vi "Q14070-B020调整螺塞压装防尘封.vi"() -> ()   [LabVIEW 2013]
uses:
  PCI8622_32.dll
panel:
  out "涂脂工步号":dbl
  out "涂脂报警提示":string
  out "换向力":dbl=2000.0 format="%#_13g"
  out "数值":i32
  out "员工ID":string
  out "型号数量":i32=10
  out "error out 4":errorcluster
  out "B020状态正常":bool
  out "B020有不合格项":bool
  out "报警提示":string
  in  "员工权限":bool=TRUE
  out "点胶工步号":dbl
  out "点胶操作状态":string
  out "涂脂操作状态":string
  out "涂脂工步号":dbl
  out "压装操作状态":string
  in  "联线按钮":bool
  out "电动缸位置(mm)":dbl format="%#_3f"
  in  "压装工步号":dbl
  out "调整螺塞压头压力(N)":dbl format="%#.1f"
  out "调整螺塞压头位移(mm)":dbl format="%#.3f"
  out "通讯状态":bool
  in  "停止":bool
  in  "选项卡控件 2":enum32{"自动", "手动", "传感器校验", "参数查询"}(tab)
  out "防尘封压装最大力(N)":dbl
  out "区域压力最大值(N)":dbl format="%#_4g"
  out "区域压力最小值(N)":dbl format="%#_4g"
  in  "压装不合格提示按钮":bool
  out "调整螺塞压防尘封":cluster{dbl[], dbl[]}[](graph)
  out "压装合格":bool
  out "压装不合格":bool
  out "压装位移(mm)":dbl format="%#_4g"
  out "监控点压力(N)":dbl format="%#_4g"
  in  "电动缸速度(s/mm)":dbl
  out "当前位置":dbl
  in  "电动缸手动位置(mm)":dbl
  in  "?":bool
  in  "防尘封涂脂":bool
  in  "手动点胶关":bool
  out "防尘封在位检测":bool
  out "涂脂在位":bool
  out "点胶在位":bool
  out "光幕":bool
  out "电动缸报警":bool
  out "电动缸原点检测":bool
  out "电动缸正极限":bool
  out "电动缸负极限":bool
  in  "M光幕无效按钮":bool
  in  "电机停止":bool
  in  "电机下降":bool
  in  "电机上升":bool
  in  "电机复位":bool
  in  "电机回原点":bool
  in  "电机使能开":bool
  in  "手动点胶开":bool
  in  "调整螺塞涂脂":bool
  in  "涂脂单循环":bool
  in  "压装单循环":bool
  in  "点胶单循环":bool
  in  "位移传感器零点偏移":dbl format="%#.2f"
  in  "位移传感器比例偏移":dbl format="%#.2f"
  in  "压力传感器零点偏移":dbl format="%#.2f"
  in  "压力传感器比例偏移":dbl format="%#.2f"
  in  "传感器参数查询":bool
  in  "传感器参数保存":bool
  in  "参数查询":bool
  in  "参数列表":string[][](table)
  in  "参数修改":bool
  out "员工姓名":string
  in  "型号选择":u16(ring) items=["J709", "J728", "J706"]
  in  "参数加载":bool
  out "报警工步号":dbl
  out "error out":errorcluster
  out "error out 2":errorcluster
  out "区域最大位移1(mm)":dbl format="%#.1f"
  out "区域最小位移1(mm)":dbl format="%#.1f"
  out "区域最大压力1(KN)":dbl format="%#.3f"
  out "位移监控点1(mm)":dbl format="%#.1f"
  out "监控点最小压力1(KN)":dbl format="%#.3f"
  out "监控点最大压力1(KN)":dbl format="%#.3f"
  out "最小压入位移1(mm)":dbl format="%#.1f"
  out "最大压入位移1(mm)":dbl format="%#.1f"
  out "区域最小压力1(KN)":dbl format="%#.3f"
  out "区域最小压力2(KN)":dbl format="%#.3f"
  out "最小压入位移2(mm)":dbl format="%#.1f"
  out "最大压入位移2(mm)":dbl format="%#.1f"
  out "区域最大压力2(KN)":dbl format="%#.3f"
  out "位移监控点2(mm)":dbl format="%#.1f"
  out "监控点最大压力2(KN)":dbl format="%#.3f"
  out "监控点最小压力2(KN)":dbl format="%#.3f"
  out "区域最小位移2(mm)":dbl format="%#.1f"
  out "区域最大位移2(mm)":dbl format="%#.1f"
  out "伺服1快进位置设置":dbl format="%#.1f"
  out "伺服1慢进位置设置":dbl format="%#.1f"
  out "压装涂脂设定次数":dbl
  out "涂脂1设定次数":dbl
  out "伺服1快进速度设置":dbl format="%#.1f"
  out "ADODB._Connection Out":refnum<k7>
  out "error out 3":errorcluster
  # "芜湖机械转向器装配线"
  # "调整螺塞压装防尘封"
  # "湖北唯思凌科装备制造有限公司 设计开发 (C)2015"
  # "Q14070机械转向器装配线"
  # "传感器校验区"
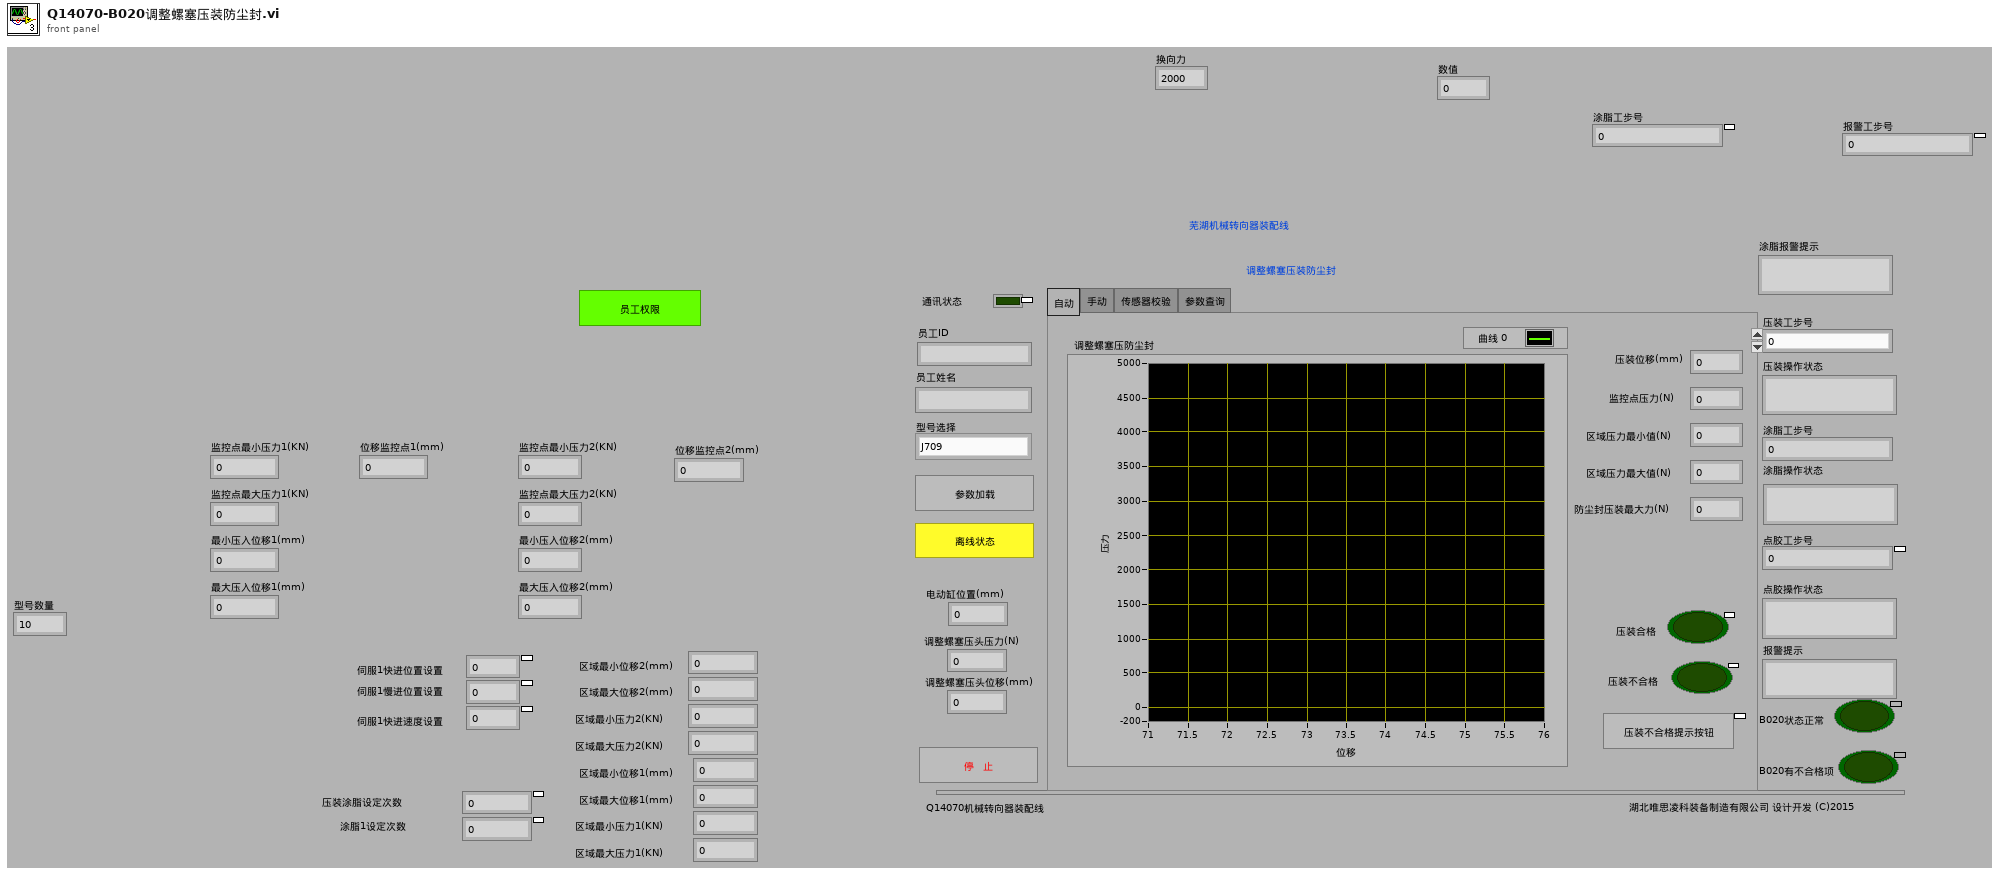
[diagram p1: front panel]
types:
  T1 = typedef "imagedata.ctl" = cluster{"image type":i32, "image depth":i32, "image":u8[], "mask":u8[], "colors":u32[], "Rectangle":cluster{"left":i16, "top":i16, "right":i16, "bottom":i16}}
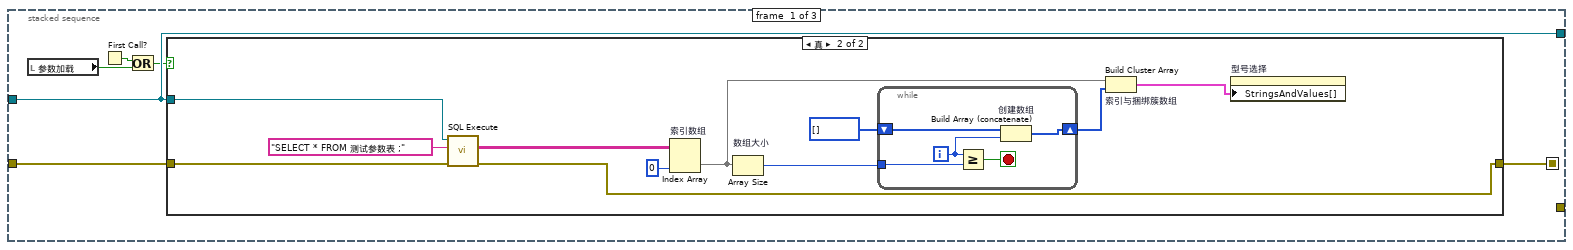
[diagram p3: hidden frame]
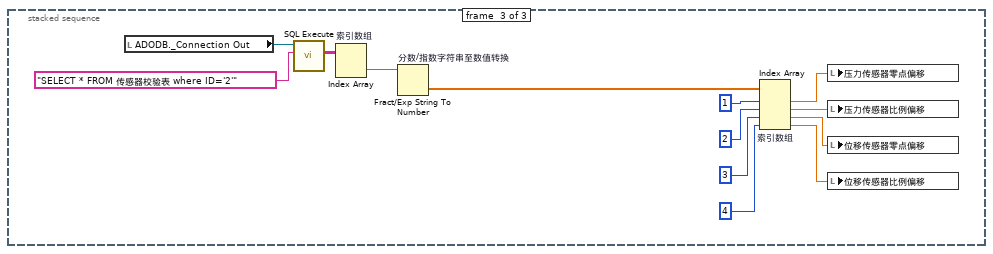
[diagram p5: hidden frame]
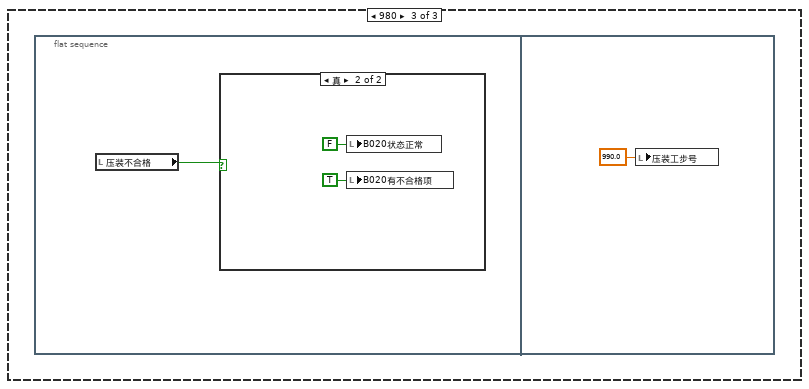
[diagram p8: hidden frame]
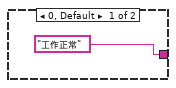
[diagram p10: hidden frame]
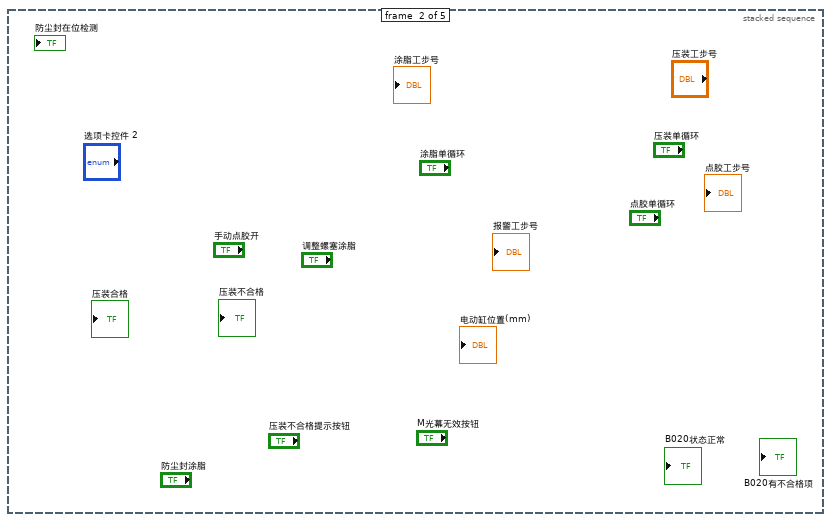
[diagram p11: hidden frame]
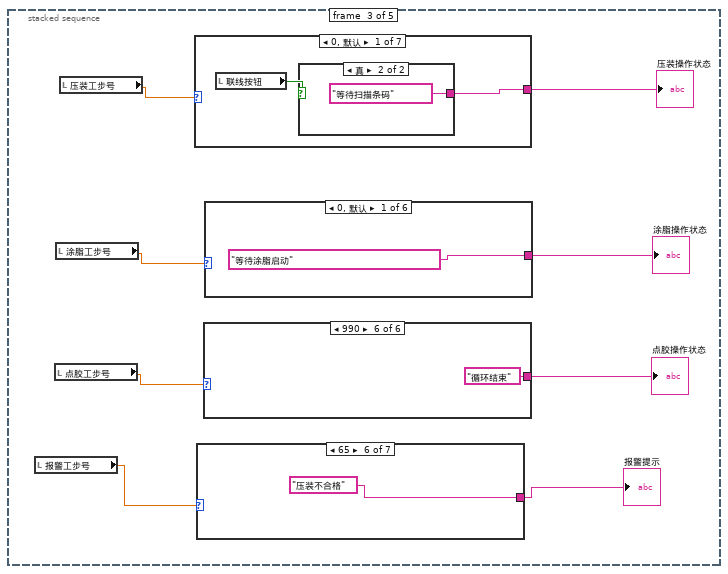
[diagram p12: hidden frame]
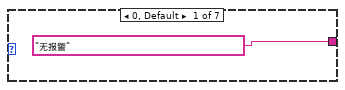
[diagram p13: hidden frame]
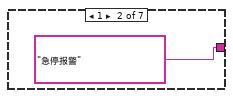
[diagram p14: hidden frame]
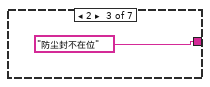
[diagram p15: hidden frame]
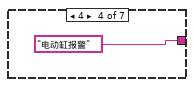
[diagram p16: hidden frame]
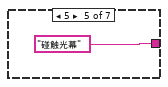
[diagram p17: hidden frame]
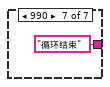
[diagram p18: hidden frame]
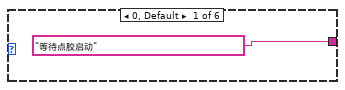
[diagram p19: hidden frame]
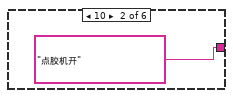
[diagram p20: hidden frame]
diagram:
  n1 = while {
    stop <- w8 stop-if-true
    n2 = event shown="[1] \"参数查询\": 值改变" {
      selector: _ -> [_ _ _ _ _]
      dyn-events: _ -> [_ _ _ _ _]
      timeout: 500 -> [_ _ _ _ _]
      event Timeout {
        n3 = event-data() -> ()  [unwired: 3 out]
      }
      event "参数查询": Value Change {
        n4 = event-data() -> ()  [unwired: 7 out]
        n5 = flat-sequence {
          tunnel: [w19] -> w16
          tunnel: [w29] -> w15
          tunnel: [w25] -> w13
          tunnel: [w22] -> w11
          tunnel: w16 -> [w34]
          tunnel: w15 -> [w32]
          tunnel: [w33] -> w14
          tunnel: w13 -> [w33]
          tunnel: [w32] -> w12
          tunnel: w11 -> [w31]
          tunnel: w14 -> [w37]
          tunnel: w12 -> [w36]
          frame #0 {
            n6 = call "字符串转换为数组.vi"("查询内容"=",产品型号,区域最小位移1,区域最大位移1,区域最小压力1,区域最大压力1,最小压入位移1,最大压入位移1,监控点最小压力1,监控点最大压力1,位移监控点1,区域最小位移2,区域最大位移2,区域最小压力2,区域最大压力2,最小压入位移2,最大压入位移2,监控点最小压力2,监控点最大压力2,位移监控点2,伺服1快进位置设置,伺服1快进速度设置,伺服1慢进位置设置,涂脂1设定次数,压装涂脂设定次数,换向压力") -> ("列首"=w17:string[])  [unwired: 10 in]
            n7 = property on="参数列表" class="Tbl (严格)"("Row Headers[]"=w17) -> ()  [unwired: 2 in, 2 out]
          }
          frame #1 {
            n8 = call "创建文本"() -> ("Result"=w30:string)  [unwired: 14 in, 1 out]
            n9 = call "ADO Connection Create.vi"() -> ("error out"=w24:errorcluster, "ADODB._Connection Out"=w28:refnum<k7>)  [unwired: 10 in]
            n10 = call "ADO Connection Open.vi"("error in (no error)"=w24, "ConnectionString"="DSN=参数B020;", "ADODB._Connection In"=w28) -> ("error out"=w23:errorcluster, "ADODB._Connection Out"=w26:refnum<k7>)  [unwired: 7 in]
            n11 = call "SQL Execute.vi"("error in (no error)"=w23, "Command Text"=w30, "ADODB._Connection In"=w26) -> ("error out"=w29:errorcluster, "Data"=w21:string[][], "ADODB._Connection Out"=w25:refnum<k7>)  [unwired: 5 in, 1 out]
            n12 = Transpose 2D Array "二维数组转置"(2D array=w21) -> (transposed array=w19:string[][])
            n13 = Index Array(array=w19, index (row)=0 ("索引 (行)")) -> (element=w22:string[])  [unwired: 1 in]
          }
          frame #2 {
            n14 = local write "参数列表"(w34) -> ()
            n15 = property on="参数列表" class="Tbl (严格)"("Column Headers[]"=w31) -> ()  [unwired: 2 in, 2 out]
          }
          frame #3 {
            n16 = call "ADO Connection Close.vi"("error in (no error)"=w36, "ADODB._Connection In"=w37) -> ("error out"=→"error out":errorcluster)  [unwired: 8 in, 1 out]
          }
        }
      }
      event "传感器参数保存": Value Change {
        n17 = event-data() -> ()  [unwired: 7 out]
        n18 = local read "压力传感器零点偏移"() -> (w41:dbl)
        n19 = local read "压力传感器比例偏移"() -> (w40:dbl)
        n20 = local read "位移传感器零点偏移"() -> (w39:dbl)
        n21 = local read "位移传感器比例偏移"() -> (w38:dbl)
        n22 = call "ADO Connection Create.vi"() -> ("error out"=w54:errorcluster, "ADODB._Connection Out"=w56:refnum<k7>)  [unwired: 10 in]
        n23 = Number To Fractional String(number=w41, precision (6)=i16 3 ("精度(6)")) -> (F-format string=w47:string)  [unwired: 2 in]
        n24 = Number To Fractional String(number=w40, precision (6)=i16 2 ("精度(6)")) -> (F-format string=w46:string)  [unwired: 2 in]
        n25 = Number To Fractional String(number=w39, precision (6)=i16 1 ("精度(6)")) -> (F-format string=w45:string)  [unwired: 2 in]
        n26 = Number To Fractional String(number=w38, precision (6)=i16 2 ("精度(6)")) -> (F-format string=w44:string)  [unwired: 2 in]
        n27 = call "创建文本2"("位移1比例偏移值"=w44, "压力1零点偏移值"=w47, "压力1比例偏移值"=w46, "位移1零点偏移值"=w45) -> ("Result"=w43:string)  [unwired: 10 in, 1 out]
        n28 = call "ADO Connection Open.vi"("error in (no error)"=w54, "ConnectionString"="DSN=参数B020;", "ADODB._Connection In"=w56) -> ("error out"=w53:errorcluster, "ADODB._Connection Out"=w55:refnum<k7>)  [unwired: 7 in]
        n29 = call "SQL Execute.vi"("error in (no error)"=w53, "Command Text"=w43, "ADODB._Connection In"=w55) -> ("error out"=w57:errorcluster, "ADODB._Connection Out"=w58:refnum<k7>)  [unwired: 5 in, 2 out]
        n30 = call "ADO Connection Close.vi"("error in (no error)"=w57, "ADODB._Connection In"=w58) -> ("error out"=→"error out 3":errorcluster)  [unwired: 8 in, 1 out]
      }
      event "停止": Value Change {
        n31 = event-data() -> ()  [unwired: 7 out]
        n32 = flat-sequence {
          frame #0 {
            n33 = local write "涂脂工步号"(0.0 ("工步号")) -> ()
          }
          frame #1 {
            n34 = Wait Until Next ms Multiple(millisecond multiple=u32 1000 ("毫秒倍数")) -> ()  [unwired: 1 out]
          }
          frame #2 {
            n35 = Quit LabVIEW(quit? (T)=TRUE ("停止？(T)")) -> ()
          }
        }
      }
      event "参数修改": Value Change {
        n36 = event-data() -> ()  [unwired: 7 out]
        n37 = while {
          i -> [w70]
          stop <- w69 stop-if-true
          (unwired) "UPDATE 测试参数表 SET 区域最小位移1='%区域最小位移1%',区域最大位移1='%区域最大位移1%',区域最小压力1='%区域最小压力1%',区域最大压力1='%区域最大压力1%', 最小压入位移1='%最小压入位移1%', 最大压入位移1='%最大压入位移1%',监控点最小压力1='%监控点最小压力1%',监控点最大压力1='%监控点最大压力1%',位移监控点1='%位移监控点1%', 区域最小位移2='%区域最小位移2%' ,区域最大位移2='%区域最大位移2%' ,区域最小压力2='%区域最小压力2%',区域最大压力2='%区域最大压力2%' ,最小压入位移2='%最小压入位移2%' ,最大压入位移2='%最大压入位移2%' ,监控点最小压力2='%监控点最小压力2%' ,监控点最大压力2='%监控点最大压力2%' ,位移监控点2='%位移监控点2%' ,伺服1快进位置设置='%伺服1快进位置设置%' ,伺服1快进速度设置='%伺服1快进速度设置%' ,伺服1慢进位置设置='%伺服1慢进位置设置%' ,伺服1慢进速度设置='%伺服1慢进速度设置%', 涂脂1设定次数='%涂脂1设定次数%'WHERE 产品型号 = '%产品型号%';"
          n38 = local read "参数列表"() -> (w72:string[][])
          n39 = local read "型号数量"() -> (w71:i32)
          n40 = Wait Until Next ms Multiple(millisecond multiple=u32 50 ("毫秒倍数")) -> ()  [unwired: 1 out]
          n41 = Greater Or Equal?(x=w70, y=w71) -> (x >= y?=w69:bool)
          n42 = Index Array(array=w72, index (col)=w70) -> (element=w68:string[])  [unwired: 1 in]
          n43 = stacked-sequence {
            seq-local: [w74 _] -> [_ w122]
            tunnel: w68 -> [w110 w129]
            tunnel: [_ w123] -> w62
            frame #0 {
              n44 = Index Array(array=w110, index #1=1 ("索引"), index #2=2 ("索引"), index #3=3 ("索引"), index #4=4 ("索引"), index #5=5 ("索引"), index #6=6 ("索引"), index #7=7 ("索引"), index #8=8 ("索引"), index #9=9 ("索引"), index #10=10 ("索引"), index #11=11 ("索引"), index #12=12 ("索引"), index #13=13 ("索引"), index #14=14 ("索引"), index #15=15 ("索引"), index #16=16 ("索引"), index #17=17 ("索引"), index #18=18 ("索引"), index #19=19 ("索引"), index #20=20 ("索引"), index #21=21 ("索引"), index #22=22 ("索引"), index #23=23 ("索引")) -> (element #1=w97:string, element #2=w96:string, element #3=w95:string, element #4=w94:string, element #5=w93:string, element #6=w92:string, element #7=w91:string, element #8=w90:string, element #9=w89:string, element #10=w88:string, element #11=w87:string, element #12=w86:string, element #13=w85:string, element #14=w84:string, element #15=w83:string, element #16=w82:string, element #17=w81:string, element #18=w80:string, element #19=w79:string, element #20=w78:string, element #21=w77:string, element #22=w76:string, element #23=w75:string)  [unwired: 1 in, 1 out]
              n45 = call "创建文本6"("区域最小位移1"=w97, "区域最大位移1"=w96, "区域最小压力1"=w95, "区域最大压力1"=w94, "最小压入位移1"=w93, "最大压入位移1"=w92, "监控点最小压力1"=w91, "监控点最大压力1"=w90, "位移监控点1"=w89, "区域最小位移2"=w88, "区域最大位移2"=w87, "区域最小压力2"=w86, "区域最大压力2"=w85, "最小压入位移2"=w84, "最大压入位移2"=w83, "监控点最小压力2"=w82, "监控点最大压力2"=w81, "位移监控点2"=w80, "伺服1快进位置设置"=w79, "伺服1快进速度设置"=w78, "伺服1慢进位置设置"=w77, "涂脂1设定次数"=w76, "压装涂脂设定次数"=w75) -> ("Result"=w74:string)  [unwired: 3 in, 1 out]
            }
            frame #1 {
              n46 = Index Array(array=w129, index #1=24, index #2=0) -> (element #1=w126:string, element #2=w125:string)  [unwired: 6 in, 6 out]
              n47 = call "创建文本5"("换向压力"=w126, "产品型号"=w125) -> ("Result"=w124:string)  [unwired: 12 in, 1 out]
              n48 = Concatenate Strings(w122, w124) -> (w123:string)
            }
          }
          n49 = local read "ADODB._Connection Out"() -> (w64:refnum<k7>)
          n50 = call "SQL Execute.vi"("error in (no error)"=errorcluster {"status"=FALSE, "code"=0, "source"=""}, "Command Text"=w62, "ADODB._Connection In"=w64) -> ("error out"=w66:errorcluster, "ADODB._Connection Out"=w67:refnum<k7>)  [unwired: 5 in, 2 out]
          n51 = call "ADO Connection Close.vi"("error in (no error)"=w66, "ADODB._Connection In"=w67) -> ("error out"=→"error out 4":errorcluster)  [unwired: 8 in, 1 out]
        }
      }
    }
    n52 = Wait Until Next ms Multiple(millisecond multiple=u32 50 ("毫秒倍数")) -> ()  [unwired: 1 out]
    n53 = local read "停止"() -> (w8:bool)
  }
  n54 = flat-sequence {
    tunnel: [w131] -> w4
    tunnel: [w130] -> w3
    tunnel: w4 -> [w138]
    tunnel: w3 -> [w137]
    tunnel: [w136] -> w2
    tunnel: [w135] -> w1
    tunnel: w2 -> [w248]
    tunnel: w1 -> [w247]
    frame #0 {
      n55 = call "ADO Connection Create.vi"() -> ("error out"=w133:errorcluster, "ADODB._Connection Out"=w134:refnum<k7>)  [unwired: 10 in]
      n56 = call "ADO Connection Open.vi"("error in (no error)"=w133, "ConnectionString"="DSN=参数B020;", "ADODB._Connection In"=w134) -> ("error out"=w130:errorcluster, "ADODB._Connection Out"=w131:refnum<k7>)  [unwired: 7 in]
      "ADODB._Connection Out" <- w131
    }
    frame #1 {
      n57 = while {
        tunnel: w138 -> [w143]
        tunnel: w137 -> [w142]
        tunnel: [w141] -> w136
        tunnel: [w140] -> w135
        stop <- w146 stop-if-true
        n58 = local read "参数加载"() -> (w139:bool)
        n59 = Wait (ms)(milliseconds to wait=u32 100 ("等待时间（毫秒）")) -> ()  [unwired: 1 out]
        n60 = First Call?() -> (First Call?: T/F=w145:bool)
        n61 = Or(x=w145, y=w139) -> (x .or. y?=w144:bool)
        n62 = case shown="真" w144 {
          tunnel: w143 -> [w149 w153]
          tunnel: w142 -> [w148 w152]
          tunnel: [w149 w151] -> w141
          tunnel: [w148 w150] -> w140
          frame False {
          }
          frame True {
            n63 = stacked-sequence {
              seq-local: [w157 _ _] -> [_ w231 _]
              tunnel: w153 -> [w158 w228 _]
              tunnel: w152 -> [w159 _ _]
              tunnel: [w158 _ _] -> w151
              tunnel: [_ w230 _] -> w150
              frame #0 {
                n64 = local read "参数加载"() -> (w155:bool)
                n65 = First Call?() -> (First Call?: T/F=w156:bool)
                n66 = Or(x=w156, y=w155) -> (x .or. y?=w154:bool)
                n67 = case shown="真" w154 {
                  tunnel: w159 -> [w160 w165]
                  tunnel: w158 -> [_ w163]
                  tunnel: [w160 w162] -> w157
                  frame False {
                  }
                  frame True {
                    n68 = call "SQL Execute.vi"("error in (no error)"=w165, "Command Text"="SELECT * FROM 测试参数表 ;", "ADODB._Connection In"=w163) -> ("error out"=w162:errorcluster, "Data"=w166:string[][])  [unwired: 5 in, 2 out]
                    n69 = Index Array "索引数组"(array=w166, index (col)=0 ("禁用的索引 (列)")) -> (element=w169:string[])  [unwired: 1 in]
                    n70 = Array Size "数组大小"(array=w169) -> (size(s)=w168:i32)
                    n71 = while {
                      shift-right: [w174] -> w167
                      shift-left: i32[] [] -> [w175]
                      tunnel: w168 -> [w172]
                      i -> [w173]
                      stop <- w176 stop-if-true
                      n72 = Greater Or Equal?(x=w173, y=w172) -> (x >= y?=w176:bool)
                      n73 = Build Array (concatenate) "创建数组"(w175, w173) -> (w174:i32[])
                    }
                    n74 = Build Cluster Array "索引与捆绑簇数组"(w169, w167) -> (w161:cluster{"String":string, i32}[])
                    n75 = property on="型号选择" class="Ring (严格)"("StringsAndValues[]"=w161) -> ()  [unwired: 2 in, 2 out]
                  }
                }
              }
              frame #1 {
                n76 = property on="型号选择" class="Ring (严格)"() -> ("RingText.Text"=w227:string)  [unwired: 2 in, 2 out]
                n77 = call "创建文本4"("产品型号"=w227) -> ("Result"=w229:string)  [unwired: 13 in, 1 out]
                n78 = call "SQL Execute.vi"("error in (no error)"=w231, "Command Text"=w229, "ADODB._Connection In"=w228) -> ("error out"=w230:errorcluster, "Data"=w233:string[][])  [unwired: 5 in, 2 out]
                n79 = Index Array "索引数组"(array=w233, index (row)=0 ("索引 (行)")) -> (element=w226:string[])  [unwired: 1 in]
                n80 = Fract/Exp String To Number "分数/指数字符串至数值转换"(string=w226) -> (number=w181:dbl[])  [unwired: 3 in, 1 out]
                n81 = Index Array(array=w181, index #1=1 ("索引"), index #2=2 ("索引"), index #3=3 ("索引"), index #4=4 ("索引"), index #5=5 ("索引"), index #6=6 ("索引"), index #7=7 ("索引"), index #8=8 ("索引"), index #9=9 ("索引"), index #10=10 ("索引"), index #11=11 ("索引"), index #12=12 ("索引"), index #13=13 ("索引"), index #14=14 ("索引"), index #15=15 ("索引"), index #16=16 ("索引"), index #17=17 ("索引"), index #18=18 ("索引"), index #19=19 ("索引"), index #20=20 ("索引"), index #21=21 ("索引"), index #22=22 ("索引"), index #23=23 ("索引"), index #24=24 ("索引")) -> (element #1=→"区域最小位移1(mm)":dbl, element #2=→"区域最大位移1(mm)":dbl, element #3=→"区域最小压力1(KN)":dbl, element #4=→"区域最大压力1(KN)":dbl, element #5=→"最小压入位移1(mm)":dbl, element #6=→"最大压入位移1(mm)":dbl, element #7=→"监控点最小压力1(KN)":dbl, element #8=→"监控点最大压力1(KN)":dbl, element #9=→"位移监控点1(mm)":dbl, element #10=→"区域最小位移2(mm)":dbl, element #11=→"区域最大位移2(mm)":dbl, element #12=→"区域最小压力2(KN)":dbl, element #13=→"区域最大压力2(KN)":dbl, element #14=→"最小压入位移2(mm)":dbl, element #15=→"最大压入位移2(mm)":dbl, element #16=→"监控点最小压力2(KN)":dbl, element #17=→"监控点最大压力2(KN)":dbl, element #18=→"位移监控点2(mm)":dbl, element #19=→"伺服1快进位置设置":dbl, element #20=→"伺服1快进速度设置":dbl, element #21=→"伺服1慢进位置设置":dbl, element #22=→"涂脂1设定次数":dbl, element #23=→"压装涂脂设定次数":dbl, element #24=→"换向力":dbl)
              }
              frame #2 {
                n82 = local read "ADODB._Connection Out"() -> (w241:refnum<k7>)
                n83 = call "SQL Execute.vi"("Command Text"="SELECT * FROM 传感器校验表 where ID='2'", "ADODB._Connection In"=w241) -> ("Data"=w246:string[][])  [unwired: 6 in, 3 out]
                n84 = Index Array "索引数组"(array=w246) -> (element=w245:string[])  [unwired: 2 in]
                n85 = Fract/Exp String To Number "分数/指数字符串至数值转换"(string=w245) -> (number=w244:dbl[])  [unwired: 3 in, 1 out]
                n86 = Index Array "索引数组"(array=w244, index #1=1 ("索引"), index #2=2 ("索引"), index #3=3 ("索引"), index #4=4 ("索引")) -> (element #1=w237:dbl, element #2=w236:dbl, element #3=w235:dbl, element #4=w234:dbl)
                n87 = local write "压力传感器零点偏移"(w237) -> ()
                n88 = local write "压力传感器比例偏移"(w236) -> ()
                n89 = local write "位移传感器零点偏移"(w235) -> ()
                n90 = local write "位移传感器比例偏移"(w234) -> ()
              }
            }
          }
        }
        n91 = local read "停止"() -> (w146:bool)
      }
    }
    frame #2 {
      n92 = call "ADO Connection Close.vi"("error in (no error)"=w247, "ADODB._Connection In"=w248) -> ("error out"=→"error out 2":errorcluster)  [unwired: 8 in, 1 out]
    }
  }
  n93 = while {
    stop <- w250 stop-if-true
    n94 = stacked-sequence {
      frame #0 {
        n95 = local read "涂脂工步号"() -> (w252:dbl)
        n96 = case shown="11" w252 {
          tunnel: ["工作正常" "涂脂报警，请加脂"] -> w253
          frame 0, Default {
          }
          frame 11 {
          }
        }
        "涂脂报警提示" <- w253
      }
      frame #1 {
      }
      frame #2 {
        n97 = local read "报警工步号"() -> (w257:dbl)
        n98 = local read "点胶工步号"() -> (w259:dbl)
        n99 = local read "涂脂工步号"() -> (w260:dbl)
        n100 = local read "压装工步号"() -> (w263:dbl)
        n101 = case shown="0, 默认" w263 {
          tunnel: [w283 "电动缸快进" ("工步操作状态") "电动缸慢进" ("工步操作状态") "开始涂脂，保持3S" ("工步操作状态") "电动缸回原点" ("工步操作状态") "压装完毕，等待复位" ("工步操作状态") "循环结束" ("工步操作状态")] -> w262
          frame 0, Default {
            n102 = local read "联线按钮"() -> (w284:bool)
            n103 = case shown="真" w284 {
              tunnel: ["等待工件" ("工步操作状态") "等待扫描条码" ("工步操作状态")] -> w283
              frame False {
              }
              frame True {
              }
            }
          }
          frame 10 {
          }
          frame 20 {
          }
          frame 30 {
          }
          frame 40 {
          }
          frame 120 {
          }
          frame 990 {
          }
        }
        "压装操作状态" <- w262
        n104 = case shown="65" w257 {
          tunnel: ["无报警" ("工步操作状态") "急停报警" ("工步操作状态") "防尘封不在位" ("工步操作状态") "电动缸报警" ("工步操作状态") "碰触光幕" ("工步操作状态") "压装不合格" ("工步操作状态") "循环结束" ("工步操作状态")] -> w256
          frame 0, Default {
          }
          frame 1 {
          }
          frame 2 {
          }
          frame 4 {
          }
          frame 5 {
          }
          frame 65 {
          }
          frame 990 {
          }
        }
        "报警提示" <- w256
        n105 = case shown="990" w259 {
          tunnel: ["等待点胶启动" ("工步操作状态") "点胶机开" ("工步操作状态") "点胶机保持" ("工步操作状态") "开始涂脂，保持3S" ("工步操作状态") "电动缸回原点" ("工步操作状态") "循环结束" ("工步操作状态")] -> w258
          frame 0, Default {
          }
          frame 10 {
          }
          frame 20 {
          }
          frame 30 {
          }
          frame 40 {
          }
          frame 990 {
          }
        }
        "点胶操作状态" <- w258
        n106 = case shown="0, 默认" w260 {
          tunnel: ["等待涂脂启动" ("工步操作状态") "开涂脂电磁阀" ("工步操作状态") "关涂脂电磁阀" ("工步操作状态") "比较涂脂阀次数" ("工步操作状态") "电动缸回原点" ("工步操作状态") "循环结束" ("工步操作状态")] -> w261
          frame 0, Default {
          }
          frame 10 {
          }
          frame 20 {
          }
          frame 30 {
          }
          frame 40 {
          }
          frame 990 {
          }
        }
        "涂脂操作状态" <- w261
      }
      frame #3 {
        n107 = First Call?() -> (First Call?: T/F=w293:bool)
        n108 = case shown="真" w293 {
          frame False {
          }
          frame True {
            n109 = call "员工管理测试程序.vi"() -> ("员工姓名"=w295:string, "员工ID"=w294:string)  [unwired: 10 in]
            n110 = local write "员工姓名"(w295) -> ()
            n111 = local write "员工ID"(w294) -> ()
          }
        }
      }
      frame #4 {
        n112 = flat-sequence {
          frame #0 {
            n113 = First Call?() -> (First Call?: T/F=w296:bool)
            n114 = case shown="假" w296 {
              frame False {
              }
              frame True {
                n115 = local write "B020有不合格项"(FALSE ("B020有不合格项")) -> ()
                n116 = local write "B020状态正常"(TRUE ("B020状态正常")) -> ()
              }
            }
          }
          frame #1 {
            n117 = while {
              stop <- w300 stop-if-true
              n118 = local read "B020有不合格项"() -> (w299:bool)
              n119 = local read "B020状态正常"() -> (w300:bool)
              n120 = case shown="假" w299 {
                frame False {
                }
                frame True {
                  n121 = call "显示对话框信息"() -> ()  [unwired: 10 in, 2 out]
                }
              }
              n122 = Wait Until Next ms Multiple(millisecond multiple=u32 50 ("毫秒倍数")) -> ()  [unwired: 1 out]
            }
          }
        }
      }
    }
    n123 = Wait Until Next ms Multiple(millisecond multiple=u32 50 ("毫秒倍数")) -> ()  [unwired: 1 out]
    n124 = local read "停止"() -> (w250:bool)
  }
  n125 = while {
    stop <- w304 stop-if-true
    n126 = local read "压装工步号"() -> (w302:dbl)
    n127 = case shown="20" w302 {
      frame 0, Default {
      }
      frame 20 {
        n128 = flat-sequence {
          tunnel: [w324] -> w321
          tunnel: [w323] -> w320
          tunnel: w321 -> [w358]
          tunnel: w320 -> [w355]
          tunnel: [w358] -> w319
          tunnel: [w355] -> w318
          tunnel: [w359] -> w317
          tunnel: w319 -> [w383]
          tunnel: w318 -> [w382]
          tunnel: w317 -> [w378]
          tunnel: [w388] -> w315
          tunnel: [w387] -> w313
          tunnel: [w386] -> w311
          tunnel: [w384] -> w308
          tunnel: ["F:\\数据存储\\"] -> w316
          tunnel: w315 -> [w399]
          tunnel: [w399] -> w314
          tunnel: w313 -> [w398]
          tunnel: [w398] -> w312
          tunnel: w311 -> [w397]
          tunnel: [w397] -> w310
          tunnel: w308 -> [w396]
          tunnel: [w396] -> w307
          tunnel: w316 -> [w413]
          tunnel: w314 -> [w412]
          tunnel: w312 -> [w411]
          tunnel: w310 -> [w410]
          tunnel: [w407] -> w309
          tunnel: w307 -> [w404]
          tunnel: [w402] -> w306
          tunnel: w309 -> [w415]
          tunnel: w306 -> [w414]
          tunnel: [w414] -> w305
          tunnel: w305 -> [w418]
          frame #0 {
            w322 = FALSE ("压装合格")
            n129 = local write "压装不合格"(w322) -> ()
            n130 = local write "压装合格"(w322) -> ()
          }
          frame #1 {
            w325 = dbl[] [] ("添加的数组")
            n131 = while {
              shift-right: [w346] -> w324
              shift-left: w325 -> [w348]
              shift-right: [w345] -> w323
              shift-left: w325 -> [w347]
              stop <- w335 stop-if-true
              (unwired) "区域2"
              (unwired) "区域1"
              n132 = local read "监控点最大压力1(KN)"() -> (w331:dbl)
              n133 = local read "监控点最小压力1(KN)"() -> (w332:dbl)
              n134 = local read "区域最大位移1(mm)"() -> (w333:dbl)
              n135 = local read "区域最小位移1(mm)"() -> (w334:dbl)
              n136 = local read "区域最大位移2(mm)"() -> (w329:dbl)
              n137 = local read "区域最小压力2(KN)"() -> (w328:dbl)
              n138 = local read "区域最大压力2(KN)"() -> (w327:dbl)
              n139 = local read "调整螺塞压头位移(mm)"() -> (w352:dbl)
              n140 = local read "区域最小位移2(mm)"() -> (w330:dbl)
              n141 = local read "调整螺塞压头压力(N)"() -> (w349:dbl)
              n142 = Multiply(x=w352, y=1.0) -> (x*y=w350:dbl)
              n143 = call "区域曲线.vi"("区域最大压力(N)"=w327, "区域最小压力(N)"=w328, "区域最大位移(mm)"=w329, "区域最小位移(mm)"=w330) -> ("区域曲线"=w339:cluster{dbl[], dbl[]})  [unwired: 7 in]
              n144 = call "区域曲线.vi"("区域最大压力(N)"=w331, "区域最小压力(N)"=w332, "区域最大位移(mm)"=w333, "区域最小位移(mm)"=w334) -> ("区域曲线"=w340:cluster{dbl[], dbl[]})  [unwired: 7 in]
              n145 = Build Array (concatenate)(w347, w349) -> (w345:dbl[])
              n146 = Build Array (concatenate)(w348, w350) -> (w346:dbl[])
              n147 = Bundle(w346, w345) -> (w344:cluster{dbl[], dbl[]})  [unwired: 1 in]
              n148 = local read "换向力"() -> (w326:dbl)
              n149 = Build Array(w344, w340, w339) -> (→"调整螺塞压防尘封":cluster{dbl[], dbl[]}[])
              n150 = Wait Until Next ms Multiple(millisecond multiple=u32 30 ("毫秒倍数")) -> ()  [unwired: 1 out]
              n151 = local read "调整螺塞压头压力(N)"() -> (w338:dbl)
              n152 = local read "压装工步号"() -> (w342:dbl)
              n153 = Greater Or Equal?(x=w342, y=30.0) -> (x >= y?=w336:bool)
              n154 = Greater Or Equal?(x=w338, y=w326) -> (x >= y?=w337:bool)
              n155 = Or(x=w337, y=w336) -> (x .or. y?=w335:bool)
            }
          }
          frame #2 {
            n156 = local read "监控点最大压力1(KN)"() -> (w370:dbl)
            n157 = local read "监控点最小压力1(KN)"() -> (w371:dbl)
            n158 = local read "区域最大位移1(mm)"() -> (w372:dbl)
            n159 = local read "区域最小位移1(mm)"() -> (w373:dbl)
            n160 = local read "最大压入位移1(mm)"() -> (w364:dbl)
            n161 = local read "最小压入位移1(mm)"() -> (w363:dbl)
            n162 = local read "位移监控点1(mm)"() -> (w368:dbl)
            n163 = Array Max & Min(array=w358) -> (max value=w369:dbl)  [unwired: 3 out]
            "压装位移(mm)" <- w369
            n164 = Wait (ms)(milliseconds to wait=u32 100 ("毫秒倍数")) -> ()  [unwired: 1 out]
            n165 = call "区域判断.vi"("压力数组"=w355, "位移数组"=w358, "区域最大压力"=w370, "区域最小压力"=w371, "区域最大位移"=w372, "区域最小位移"=w373) -> ("数值 2"=→"区域压力最小值(N)":dbl, "数值"=→"区域压力最大值(N)":dbl, "区域监控合格"=w360:bool)  [unwired: 1 in]
            n166 = call "压力位移插值.vi"("压力数组"=w355, "监控点位移"=w368, "位移数组"=w358) -> ("监控点压力"=w367:dbl)  [unwired: 2 in]
            "监控点压力(N)" <- w367
            n167 = local read "监控点最小压力1(KN)"() -> (w365:dbl)
            n168 = local read "监控点最大压力1(KN)"() -> (w366:dbl)
            n169 = In Range and Coerce(upper limit=w364, x=w369, lower limit=w363) -> (In Range?=w361:bool)  [unwired: 1 out]
            n170 = Array Max & Min(array=w355) -> (max value=→"防尘封压装最大力(N)":dbl)  [unwired: 3 out]
            n171 = In Range and Coerce(upper limit=w366, x=w367, lower limit=w365) -> (In Range?=w362:bool)  [unwired: 1 out]
            n172 = Compound Arithmetic op=AND(w362, w361, w360) -> (w359:bool)
          }
          frame #3 {
            (unwired) "数据存储"
            n173 = Build Array(w383, w382) -> (w381:dbl[][])
            n174 = Not(x=w378) -> (.not. x?=w377:bool)
            n175 = local read "数值"() -> (w375:i32)
            n176 = call "数据存储.vi"("字符串"="E:\\sjcc\\", "2D data"=w381) -> ()  [unwired: 10 in]
            n177 = Wait (ms)(milliseconds to wait=u32 200 ("等待时间（毫秒）")) -> ()  [unwired: 1 out]
            n178 = local write "压装不合格"(w377) -> ()
            n179 = local write "压装合格"(w378) -> ()
            n180 = Increment(x=w375) -> (x+1=→"数值":i32)
          }
          frame #4 {
            n181 = local read "数值"() -> (w384:i32)
            n182 = Format Date/Time String(time format string (%c)="%Y%m%d") -> (date/time string=w385:string)  [unwired: 2 in]
            n183 = String Subset(string=w385, offset (0)=4 ("偏移量(0)"), length (rest)=2 ("长度（剩余）")) -> (substring=w387:string)
            n184 = String Subset(string=w385, offset (0)=6 ("偏移量(0)"), length (rest)=2 ("长度（剩余）")) -> (substring=w386:string)
            n185 = String Subset(string=w385, offset (0)=0 ("偏移量(0)"), length (rest)=4 ("长度（剩余）")) -> (substring=w388:string)
          }
          frame #5 {
          }
          frame #6 {
            w409 = "\\"
            n186 = Number To Decimal String(number=w404) -> (decimal integer string=w405:string)  [unwired: 1 in]
            n187 = Concatenate Strings(w413, w412, w409, w411, w409, w410, w409) -> (w408:string)
            n188 = Concatenate Strings(w413, w412, w409, w411, w409, w410, w409) -> (w406:string)
            n189 = Concatenate Strings(w406, w405, ".JPG" ("字符串")) -> (w401:string)
            n190 = String To Path(string=w408) -> (path=w407:path)
            n191 = String To Path(string=w401) -> (path=w402:path)
          }
          frame #7 {
            n192 = call <vilib>:"Check if File or Folder Exists.vi"("path"=w415) -> ("file or folder exists?"=w416:bool)  [unwired: 8 in, 2 out]
            n193 = case shown="假" w416 {
              tunnel: w415 -> [w417 _]
              frame False {
                n194 = Create Folder(path (use dialog)=w417) -> ()  [unwired: 2 in, 3 out]
              }
              frame True {
              }
            }
          }
          frame #8 {
            n195 = control-ref of="本VI"() -> (w420:refnum<vi>)
            n196 = invoke class="VI" method="FP.Get Image"(reference=w420) -> ("image data"=w419:T1)  [unwired: 5 in, 5 out]
            n197 = call <vilib>:"Write JPEG File.vi"("image data"=w419, "path to JPEG file"=w418) -> ()  [unwired: 8 in, 2 out]
          }
          frame #9 {
            n198 = local write "压装工步号"(40.0 ("压装工步号")) -> ()
          }
        }
      }
      frame 980 {
        n199 = flat-sequence {
          frame #0 {
            n200 = local read "压装不合格"() -> (w422:bool)
            n201 = case shown="真" w422 {
              frame False {
              }
              frame True {
                n202 = local write "B020状态正常"(FALSE ("B020状态正常")) -> ()
                n203 = local write "B020有不合格项"(TRUE ("B020有不合格项")) -> ()
              }
            }
          }
          frame #1 {
            n204 = local write "压装工步号"(990.0 ("压装工步号")) -> ()
          }
        }
      }
    }
    n205 = Wait Until Next ms Multiple(millisecond multiple=u32 50 ("毫秒倍数")) -> ()  [unwired: 1 out]
    n206 = local read "停止"() -> (w304:bool)
  }
  n207 = flat-sequence {
    tunnel: [w426] -> w7
    tunnel: w7 -> [w428]
    tunnel: [w427] -> w6
    tunnel: w6 -> [w469]
    tunnel: [w469] -> w5
    tunnel: w5 -> [w471]
    frame #0 {
      n208 = call "PCI8622配置.vi"() -> ("DeviceID"=w426:i32)  [unwired: 11 in]
    }
    frame #1 {
      n209 = while {
        tunnel: w428 -> [w456]
        tunnel: [w456] -> w427
        stop <- "停止" stop-if-true
        w466 = 0  # nRetSizeWords
        w467 = 2048  # nReadSizeWords
        # "hDevice"
        n210 = Initialize Array(u16 0, 2048 ("dimension size")) -> (w457:u16[])
        n211 = local read "电动缸位置(mm)"() -> (→"当前位置":dbl)
        n212 = dll-call lib="PCI8622_32.dll" fn="PCI8622_ReadDeviceProAD_Npt" label="ReadDeviceProAD_Npt"("hDevice"=w456, "ADBuffer[]"=w457, "nReadSizeWords"=w467, "nRetSizeWords"=w466) -> ("ADBuffer[]"=w460:u16[])  [unwired: 7 in, 2 out]
        n213 = Divide(x=w460, y=65536.01) -> (x/y=w461:dbl[])
        n214 = Multiply(x=w461, y=20) -> (x*y=w464:dbl[])
        n215 = Subtract(x=w464, y=10) -> (x-y=w450:dbl[])
        n216 = Decimate 1D Array "抽取一维数组"(w450) -> (w431:dbl[], w430:dbl[])  [unwired: 6 out]
        n217 = Add Array Elements(numeric array=w430) -> (sum=w451:dbl)
        n218 = Add Array Elements(numeric array=w431) -> (sum=w454:dbl)
        n219 = Array Size(array=w430) -> (size(s)=w452:i32)
        n220 = Array Size(array=w431) -> (size(s)=w453:i32)
        n221 = Divide(x=w451, y=w452) -> (x/y=w447:dbl)
        n222 = Divide(x=w454, y=w453) -> (x/y=w448:dbl)
        n223 = local read "位移传感器零点偏移"() -> (w435:dbl)
        n224 = local read "位移传感器比例偏移"() -> (w434:dbl)
        n225 = Multiply(x=25.0 ("y"), y=w448) -> (x*y=w436:dbl)
        n226 = Subtract(x=w447, y=-0.53) -> (x-y=w445:dbl)
        n227 = local read "压力传感器零点偏移"() -> (w440:dbl)
        n228 = local read "压力传感器比例偏移"() -> (w438:dbl)
        n229 = Multiply(x=w445, y=500.0) -> (x*y=w443:dbl)
        n230 = Subtract(x=w436, y=w435) -> (x-y=w433:dbl)
        n231 = Multiply(x=w433, y=w434) -> (x*y=→"调整螺塞压头位移(mm)":dbl)
        n232 = Add(x=w443, y=0.0) -> (x+y=w441:dbl)
        n233 = Subtract(x=w441, y=w440) -> (x-y=w439:dbl)
        n234 = Multiply(x=w439, y=w438) -> (x*y=→"调整螺塞压头压力(N)":dbl)
        n235 = Wait Until Next ms Multiple(millisecond multiple=u32 20 ("毫秒倍数")) -> ()  [unwired: 1 out]
      }
    }
    frame #2 {
      n236 = dll-call lib="PCI8622_32.dll" fn="PCI8622_StopDeviceProAD" label="StopDeviceProAD"("hDevice"=w469) -> ("hDevice"=w470:i32)  [unwired: 4 in, 2 out]
      n237 = dll-call lib="PCI8622_32.dll" fn="PCI8622_ReleaseDeviceProAD" label="ReleaseDeviceProAD"("hDevice"=w470) -> ()  [unwired: 5 in, 2 out]
    }
    frame #3 {
      n238 = dll-call lib="PCI8622_32.dll" fn="PCI8622_ReleaseDevice" label="ReleaseDevice"("hDevice"=w471) -> ()  [unwired: 5 in, 2 out]
    }
  }
